vi "test Get-Set-Get Parameter Definitions.vi"(8 "error in":errorcluster, 11 "TestCase in":refnum<class "Scripting.lvclass">) -> (0 "error out":errorcluster, 3 "TestCase out":refnum<class "Scripting.lvclass">)   [LabVIEW 2020, in "Scripting.lvclass"]
uses:
  Scripting.lvclass
  Shared/Parameter Definition.ctl
  Encoding and Decoding/Encoding.ctl
  Scripting.lvclass/Scripting.ctl
  Scripting/Constants.vi
  <vilib>/NI VeriStand/Custom Device Tools/Custom Device Utility Library/NI VeriStand - Search for Item by GUID.vi
  <vilib>/addons/_JKI Toolkits/VI Tester/TestCase.llb/TestCase.lvclass
  Scripting/Ballard ARINC 429 Scripting.lvlib
  Encoding and Decoding/Encoding and Decoding.lvlib
  <vilib>/NI VeriStand/Custom Device Tools/Custom Device Utility Library/Custom Device Utility Library.lvlib
  <vilib>/NI VeriStand/Custom Device API/Custom Device API.lvlib
  C:/Program Files (x86)/National Instruments/LabVIEW 2020/vi.lib/addons/_JKI Toolkits/VI Tester/TestCase.llb/TestCase.lvclass
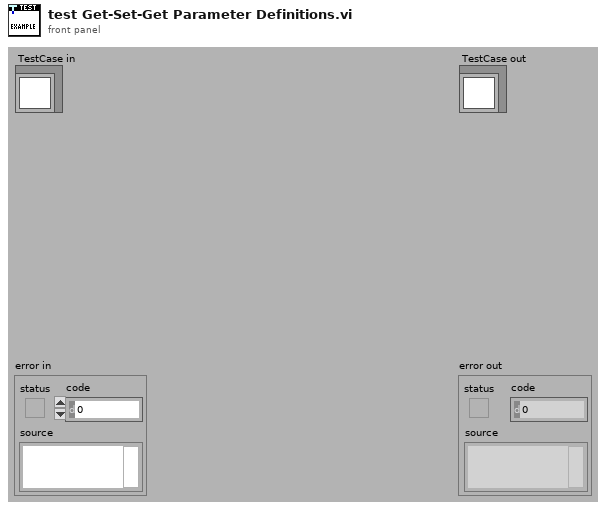
[diagram p1: front panel]
types:
  T1 = typedef "Parameter Definition.ctl" = cluster{"start index":i32, "size":i32, "encoding":T2, "signed":bool, "scale multiplier":dbl, "scale offset":dbl}
  T2 = typedef "Encoding and Decoding.lvlib/Encoding.ctl" = enum16{"BNR", "BCD", "Discrete"}
  T3 = typedef "Custom Device API.lvlib/Custom Device Item Ref.ctl" = u64
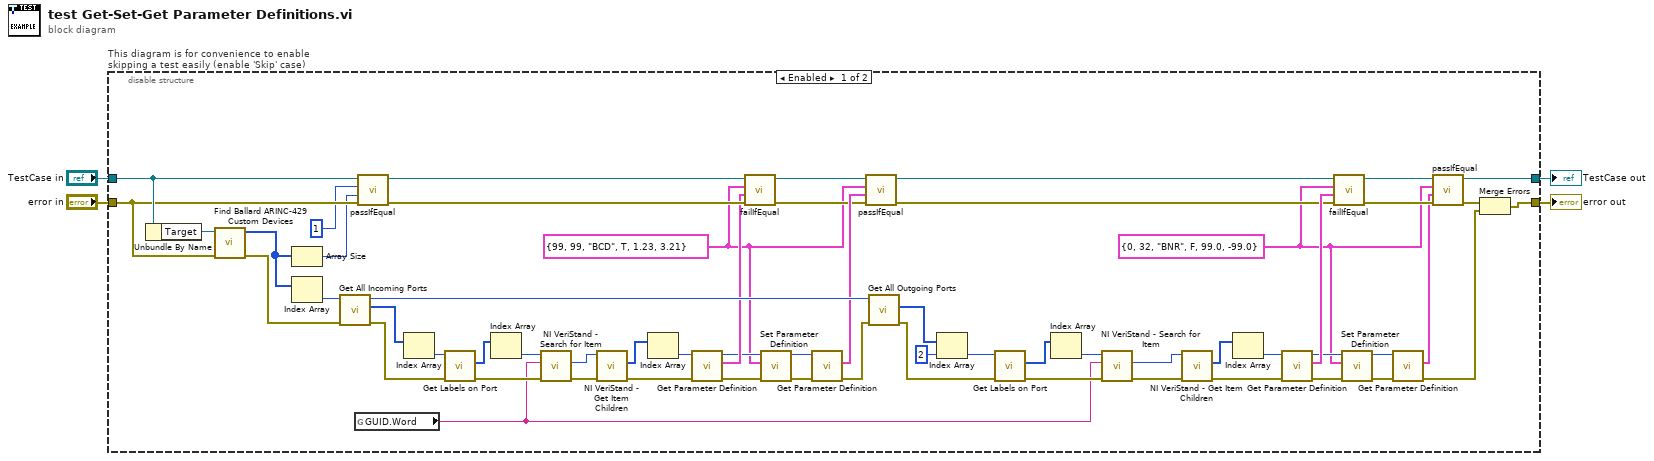
[diagram p0: block diagram]
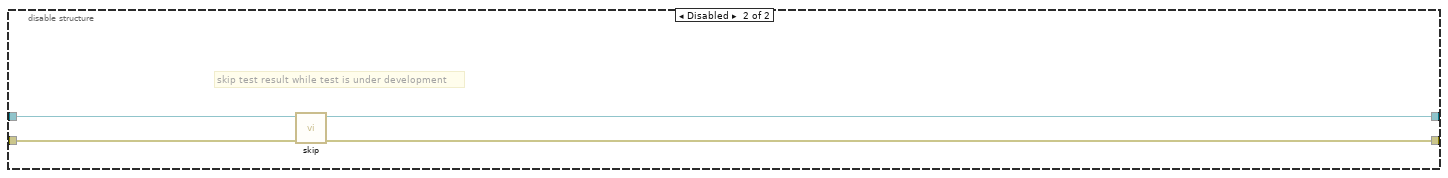
[diagram p2: hidden frame]
diagram:
  n1 = disable-structure "This diagram is for convenience to enable skipping a test easily (enable 'Skip' case)" shown="Enabled" {
    disable-tunnel: "TestCase in" -> [w62 w68]
    disable-tunnel: [w7 w66] -> w1
    disable-tunnel: [w50 w67] -> w3
    disable-tunnel: "error in" -> [w61 w65]
    frame Enabled {
      w16 = T1 {"start index"=99, "size"=99, "encoding"=enum."BCD", "signed"=TRUE, "scale multiplier"=1.23, "scale offset"=3.21} ("parameter definition")
      w5 = T1 {"start index"=0, "size"=32, "encoding"=enum."BNR", "signed"=FALSE, "scale multiplier"=99.0, "scale offset"=-99.0} ("parameter definition")
      n2 = Unbundle By Name(w62) -> ("Target"=w64:refnum<k24>)
      n3 = call "Find Ballard ARINC-429 Custom Devices.vi"("error in"=w61, "target"=w64) -> ("error out"=w54:errorcluster, "Ballard ARINC-429 custom devices"=w60:u64[])  [unwired: 8 in]
      n4 = Array Size(array=w60) -> (size(s)=w58:i32)
      n5 = Index Array(array=w60) -> (element=w63:u64)  [unwired: 1 in]
      n6 = call "Get All Incoming Ports.vi"("error in"=w54, "Ballard ARINC 429 ref"=w63) -> ("error out"=w47:errorcluster, "Port refs"=w57:T3[], "Ballard ARINC 429 ref out"=w53:T3)  [unwired: 7 in]
      n7 = global read "Constants.vi" "GUID.Word"() -> (w27:string)
      n8 = call-dynamic "passIfEqual.vi"("error in (no error)"=w61, "y"=w58, "x"=1 ("size(s)"), "TestCase in"=w62) -> ("error out"=w55:errorcluster, "TestCase out"=w56:refnum<class "Scripting.lvclass">)  [unwired: 6 in]
      n9 = Index Array(array=w57) -> (element=w48:T3)  [unwired: 1 in]
      n10 = call "Get Labels on Port.vi"("error in"=w47, "port ref"=w48) -> ("error out"=w28:errorcluster, "label references"=w30:T3[])  [unwired: 6 in, 2 out]
      n11 = Index Array(array=w30) -> (element=w29:T3)  [unwired: 1 in]
      n12 = call-poly <vilib>:"NI VeriStand - Search for Item.vi"("error in"=w28, "Item GUID"=w27, "Section Ref in"=w29) -> ("error out"=w35:errorcluster, "Item Ref"=w34:T3)  [unwired: 5 in, 2 out]
      n13 = call <vilib>:"NI VeriStand - Get Item Children.vi"("error in (no error)"=w35, "Item Ref in"=w34) -> ("error out"=w32:errorcluster, "Child Refs"=w36:T3[])  [unwired: 6 in, 2 out]
      n14 = Index Array(array=w36) -> (element=w33:T3)  [unwired: 1 in]
      n15 = call "Get Parameter Definition.vi"("error in"=w32, "parameter ref in"=w33) -> ("error out"=w26:errorcluster, "parameter definition"=w31:T1, "parameter ref out"=w25:T3)  [unwired: 7 in]
      n16 = call-dynamic "failIfEqual.vi"("error in (no error)"=w55, "y"=w31, "x"=w16, "TestCase in"=w56) -> ("error out"=w20:errorcluster, "TestCase out"=w19:refnum<class "Scripting.lvclass">)  [unwired: 6 in]
      n17 = call "Set Parameter Definition.vi"("error in"=w26, "parameter definition"=w16, "parameter ref in"=w25) -> ("error out"=w24:errorcluster, "parameter ref out"=w23:T3)  [unwired: 7 in]
      n18 = call "Get Parameter Definition.vi"("error in"=w24, "parameter ref in"=w23) -> ("error out"=w22:errorcluster, "parameter definition"=w21:T1)  [unwired: 7 in, 1 out]
      n19 = call-dynamic "passIfEqual.vi"("error in (no error)"=w20, "y"=w21, "x"=w16, "TestCase in"=w19) -> ("error out"=w18:errorcluster, "TestCase out"=w17:refnum<class "Scripting.lvclass">)  [unwired: 6 in]
      n20 = call "Get All Outgoing Ports.vi"("error in"=w22, "Ballard ARINC 429 ref"=w53) -> ("error out"=w46:errorcluster, "Port refs"=w52:T3[])  [unwired: 7 in, 1 out]
      n21 = Index Array(array=w52, index=2) -> (element=w45:T3)
      n22 = call "Get Labels on Port.vi"("error in"=w46, "port ref"=w45) -> ("error out"=w42:errorcluster, "label references"=w44:T3[])  [unwired: 6 in, 2 out]
      n23 = Index Array(array=w44) -> (element=w43:T3)  [unwired: 1 in]
      n24 = call-poly <vilib>:"NI VeriStand - Search for Item.vi"("error in"=w42, "Item GUID"=w27, "Section Ref in"=w43) -> ("error out"=w40:errorcluster, "Item Ref"=w41:T3)  [unwired: 5 in, 2 out]
      n25 = call <vilib>:"NI VeriStand - Get Item Children.vi"("error in (no error)"=w40, "Item Ref in"=w41) -> ("error out"=w39:errorcluster, "Child Refs"=w37:T3[])  [unwired: 6 in, 2 out]
      n26 = Index Array(array=w37) -> (element=w38:T3)  [unwired: 1 in]
      n27 = call "Get Parameter Definition.vi"("error in"=w39, "parameter ref in"=w38) -> ("error out"=w13:errorcluster, "parameter definition"=w49:T1, "parameter ref out"=w12:T3)  [unwired: 7 in]
      n28 = call-dynamic "failIfEqual.vi"("error in (no error)"=w18, "y"=w49, "x"=w5, "TestCase in"=w17) -> ("error out"=w10:errorcluster, "TestCase out"=w8:refnum<class "Scripting.lvclass">)  [unwired: 6 in]
      n29 = call "Set Parameter Definition.vi"("error in"=w13, "parameter definition"=w5, "parameter ref in"=w12) -> ("error out"=w14:errorcluster, "parameter ref out"=w15:T3)  [unwired: 7 in]
      n30 = call "Get Parameter Definition.vi"("error in"=w14, "parameter ref in"=w15) -> ("error out"=w11:errorcluster, "parameter definition"=w6:T1)  [unwired: 7 in, 1 out]
      n31 = call-dynamic "passIfEqual.vi"("error in (no error)"=w10, "y"=w6, "x"=w5, "TestCase in"=w8) -> ("error out"=w9:errorcluster, "TestCase out"=w7:refnum<class "Scripting.lvclass">)  [unwired: 6 in]
      n32 = Merge Errors(w9, w11) -> (w50:errorcluster)
    }
    frame Disabled {
      # "skip test result while test is under development"
      n33 = call <vilib>:"skip.vi"("error in (no error)"=w65, "TestCase in"=w68) -> ("error out"=w67:errorcluster, "TestCase out"=w66:refnum<class "Scripting.lvclass">)  [unwired: 8 in]
    }
  }
  "error out" <- w3
  "TestCase out" <- w1
